vi "Add Result Sections.vi"(8 "error in":errorcluster, 10 "WaveformTask ID":T1 format="%.0x", 11 "CustomDevice Ref":T1 format="%.0x") -> (0 "error out":errorcluster, 3 "CustomDevice Ref":T1 format="%.0x")   [LabVIEW 2014, in "Waveform-Processing-Custom-Device System Explorer.lvlib"]
uses:
  Waveform-Processing-Custom-Device System Explorer.lvlib
  <vilib>/NI Veristand/Custom Device API/Custom Device Item Ref.ctl
  NationalInstruments.VeriStand.SystemStorage
  Shared/Constants.vi
  <vilib>/NI Veristand/Custom Device API/Set Item Property (Dependent Node Pointer).vi
  <vilib>/NI Veristand/Custom Device Tools/Custom Device Utility Library/Custom Device Utility Library.lvlib
  <vilib>/NI Veristand/Custom Device API/Custom Device API.lvlib
  Shared/Waveform-Processing-Custom-Device Shared.lvlib
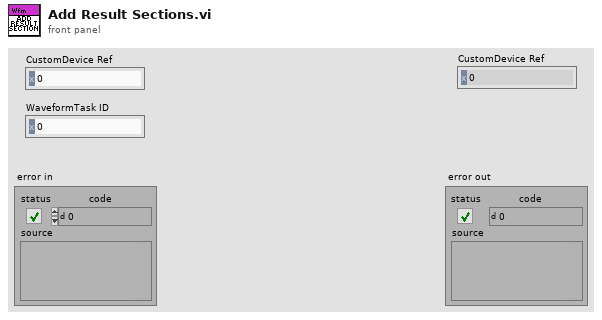
[diagram p1: front panel]
types:
  T1 = typedef "Custom Device API.lvlib/Custom Device Item Ref.ctl" = u64
  T2 = typedef "Custom Device API.lvlib/Custom Device Pointer.ctl" = refnum<k24>
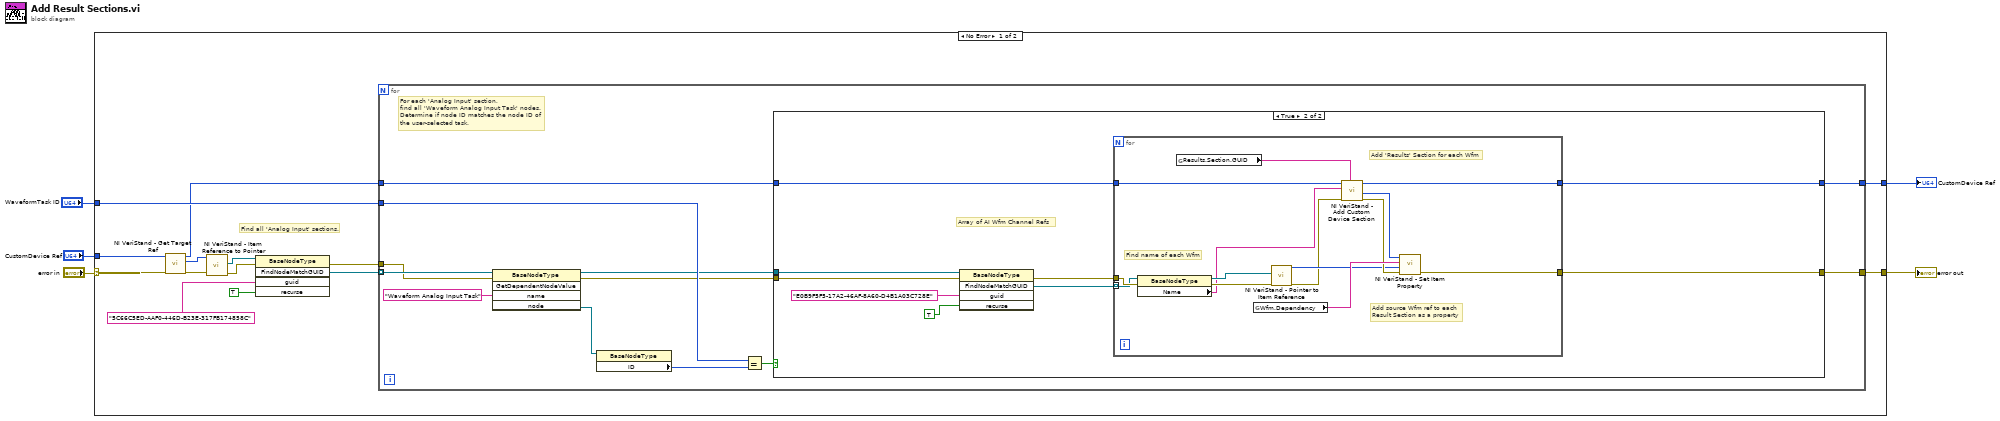
[diagram p0: block diagram]
diagram:
  n1 = case shown="No Error" "error in" {
    selector: "error in" -> [w19 w58]
    tunnel: [w7 w58] -> w4
    tunnel: "CustomDevice Ref" -> [w18 w57]
    tunnel: "WaveformTask ID" -> [w17 _]
    tunnel: [w6 w57] -> w1
    frame No Error {
      # "Find all 'Analog Input' sections."
      n2 = call <vilib>:"NI VeriStand - Get Target Ref.vi"("error in"=w19, "Item Ref in"=w18) -> ("error out"=w15:errorcluster, "Target Ref"=w14:T1, "Item Ref out"=w16:T1)  [unwired: 6 in, 1 out]
      n3 = call <vilib>:"NI VeriStand - Item Reference to Pointer.vi"("error in (no error)"=w15, "Item Ref in"=w14) -> ("error out"=w12:errorcluster, "Node Pointer"=w13:T2)  [unwired: 6 in, 2 out]
      n4 = invoke class="BaseNodeType" method="FindNodeMatchGUID"(reference=w13, error in=w12, "guid"="5C66C5ED-AAF0-446D-B23E-317FB174858C" ("Item GUID"), "recurse"=TRUE ("Find All? (T)")) -> (error out=w8:errorcluster, "FindNodeMatchGUID"=w9:refnum<k24>[])  [unwired: 1 in, 3 out]
      n5 = for {
        tunnel: w17 -> [w31]
        tunnel: w16 -> [w22]
        tunnel: w9 -> [w30] mode=indexing
        tunnel: w8 -> [w29]
        tunnel: [w21] -> w7
        tunnel: [w20] -> w6
        # "For each 'Analog Input' section, \nfind all 'Waveform Analog Input Task' nodes.\nDetermine if node ID matches the node ID of \nthe user-selected task."
        n6 = invoke class="BaseNodeType" method="GetDependentNodeValue"(reference=w30, error in=w29, "name"="Waveform Analog Input Task" ("Property Name")) -> (reference out=w25:refnum<k24>, error out=w24:errorcluster, "node"=w27:refnum<k24>)  [unwired: 2 in, 2 out]
        n7 = property class="BaseNodeType"(reference=w27) -> ("ID"=w26:u64)  [unwired: 1 in, 2 out]
        n8 = Equal?(x=w31, y=w26) -> (x = y?=w23:bool)
        n9 = case shown="True" w23 {
          tunnel: w25 -> [_ w42]
          tunnel: w24 -> [w33 w40]
          tunnel: w22 -> [w32 w37]
          tunnel: [w33 w35] -> w21
          tunnel: [w32 w34] -> w20
          frame False {
          }
          frame True {
            # "Array of AI Wfm Channel Refs"
            n10 = invoke class="BaseNodeType" method="FindNodeMatchGUID"(reference=w42, error in=w40, "guid"="E0B9F5F5-17A2-46AF-8A60-D4B1A03C728E", "recurse"=TRUE ("Find All? (T)")) -> (error out=w36:errorcluster, "FindNodeMatchGUID"=w38:refnum<k24>[])  [unwired: 1 in, 3 out]
            n11 = for {
              tunnel: w38 -> [w54] mode=indexing
              tunnel: w37 -> [w56]
              tunnel: w36 -> [w55]
              tunnel: [w47] -> w35
              tunnel: [w43] -> w34
              # "Find name of each Wfm"
              # "Add 'Results' Section for each Wfm"
              # "Add source Wfm ref to each\nResult Section as a property"
              n12 = property class="BaseNodeType"(reference=w54, error in=w55) -> (reference out=w51:refnum<k24>, error out=w49:errorcluster, "Name"=w45:string)
              n13 = global read "Constants.vi" "Results.Section.GUID"() -> (w44:string)
              n14 = global read "Constants.vi" "Wfm.Dependency"() -> (w53:string)
              n15 = call <vilib>:"NI VeriStand - Pointer to Item Reference.vi"("error in (no error)"=w49, "Node Pointer"=w51) -> ("error out"=w48:errorcluster, "Item Ref out"=w50:T1)  [unwired: 8 in]
              n16 = call <vilib>:"NI VeriStand - Add Custom Device Section.vi"("GUID (Default Section)"=w44, "error in (no error)"=w48, "Section Name"=w45, "Parent Ref in"=w56) -> ("error out"=w52:errorcluster, "Section Ptr"=w46:T1, "Parent Ref out"=w43:T1)  [unwired: 4 in, 1 out]
              n17 = call-poly <vilib>:"NI VeriStand - Set Item Property.vi"("error in (no error)"=w52, "Dependent Node Ref"=w50, "Property Name"=w53, "Item Ref in"=w46) -> ("error out"=w47:errorcluster)  [unwired: 5 in, 2 out]
            }
          }
        }
      }
    }
    frame Error {
    }
  }
  "error out" <- w4
  "CustomDevice Ref" <- w1
